vi "Scripting_UpdateGoop2Create.vi"(0 "ViRef":refnum<vi>, 1 "RemovePreloadDynamicMethods":bool, 5 "error in (no error)":errorcluster) -> (19 "error out":errorcluster)   [LabVIEW 2020]
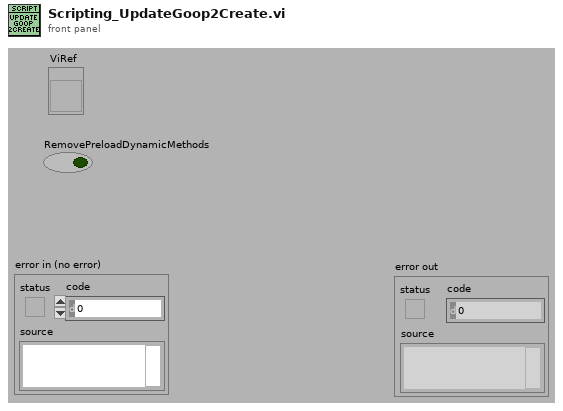
[diagram p1: front panel]
types:
  T1 = cluster{"OORefControls":refnum<vi>[], "ClassOORefs":path[], "ParentClassCreateVI":path}
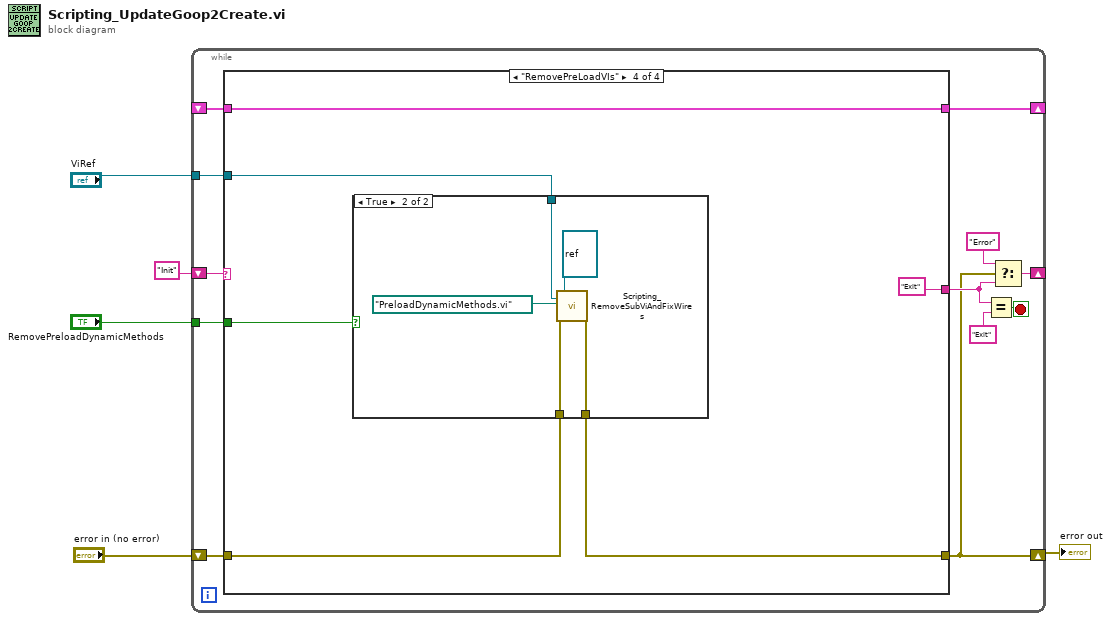
[diagram p0: block diagram]
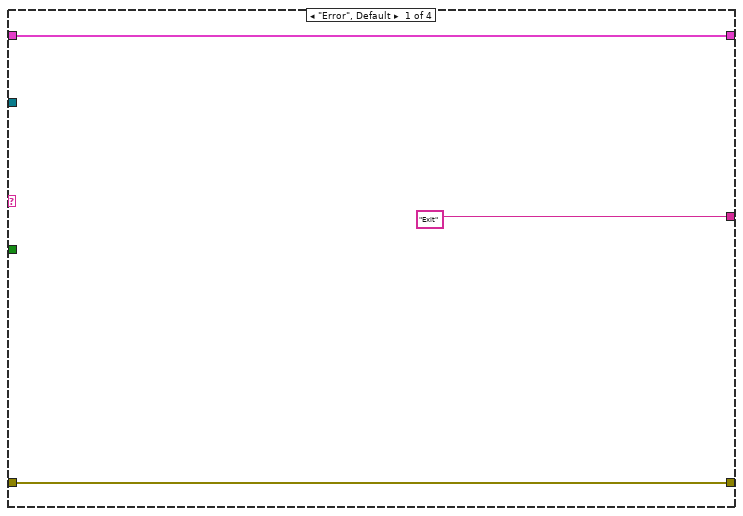
[diagram p2: hidden frame]
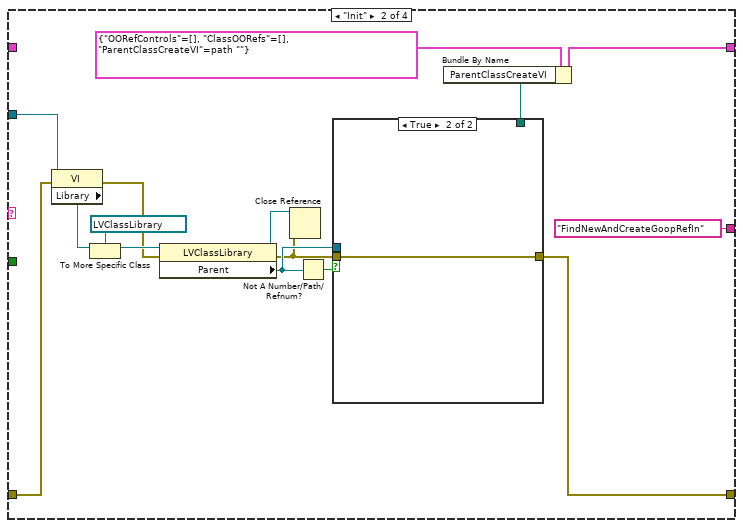
[diagram p3: hidden frame]
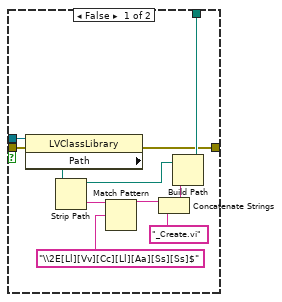
[diagram p4: hidden frame]
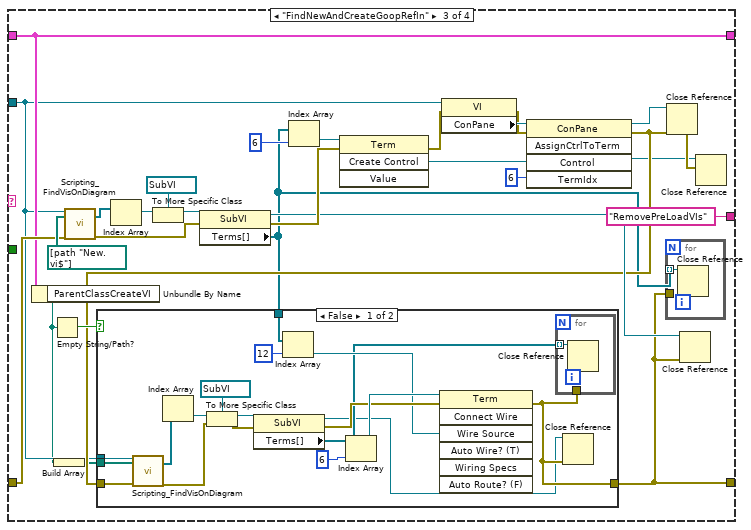
[diagram p5: hidden frame]
diagram:
  n1 = while {
    shift-right: [w10] -> w3
    shift-left: "error in (no error)" -> [w17]
    shift-right: [w15] -> _
    shift-left: "Init" -> [w16]
    shift-right: [w9] -> _
    shift-left: _ -> [w8]
    tunnel: "ViRef" -> [w7]
    tunnel: "RemovePreloadDynamicMethods" -> [w6]
    stop <- w14 stop-if-true
    n2 = case shown="\"RemovePreLoadVIs\"" w16 {
      tunnel: w17 -> [w20 w32 w59 w101]
      tunnel: [w20 w21 w55 w99] -> w10
      tunnel: ["Exit" "FindNewAndCreateGoopRefIn" "RemovePreLoadVIs" "Exit"] -> w11
      tunnel: [w18 w26 w58 w98] -> w9
      tunnel: w8 -> [w18 _ w58 w98]
      tunnel: w7 -> [_ w34 w53 w100]
      tunnel: w6 -> [_ _ _ w96]
      frame "Error", Default {
      }
      frame "Init" {
        n3 = property class="VI"(reference=w34, error in=w32) -> (error out=w28:errorcluster, "Library"=w31:refnum<vi>)  [unwired: 1 out]
        n4 = To More Specific Class(target class=refnum<vi> refnum ("LVClassLibrary Refnum"), reference=w31) -> (specific class reference=w29:refnum<vi>)  [unwired: 1 in, 1 out]
        n5 = property class="LVClassLibrary"(reference=w29, error in=w28) -> (reference out=w23:refnum<vi>, error out=w24:errorcluster, "Parent"=w25:refnum<vi>)
        n6 = Close Reference(reference=w23, error in (no error)=w24) -> ()  [unwired: 1 out]
        n7 = Not A Number/Path/Refnum?(number/path/refnum=w25) -> (NaN/Path/Refnum?=w33:bool)
        n8 = case shown="True" w33 {
          tunnel: w24 -> [w46 w47]
          tunnel: w25 -> [w45 _]
          tunnel: [w37 _] -> w22
          tunnel: [w36 w47] -> w21
          frame False {
            n9 = property class="LVClassLibrary"(reference=w45, error in=w46) -> (error out=w36:errorcluster, "Path"=w44:path)  [unwired: 1 out]
            n10 = Strip Path(path=w44) -> (stripped path=w38:path, name=w42:string)
            n11 = Match Pattern(string=w42, regular expression="\\2E[Ll][Vv][Cc][Ll][Aa][Ss][Ss]$") -> (before substring=w41:string)  [unwired: 1 in, 3 out]
            n12 = Concatenate Strings(w41, "_Create.vi" ("string")) -> (w39:string)
            n13 = Build Path(base path=w38, name or relative path=w39) -> (appended path=w37:path)
          }
          frame True {
          }
        }
        n14 = Bundle By Name(cluster=T1 {"OORefControls"=[], "ClassOORefs"=[], "ParentClassCreateVI"=path ""}, "ParentClassCreateVI"=w22) -> (w26:T1)
      }
      frame "FindNewAndCreateGoopRefIn" {
        n15 = Unbundle By Name(w58) -> ("ParentClassCreateVI"=w52:path)
        n16 = Empty String/Path?(string/path=w52) -> (empty?=w57:bool)
        n17 = Build Array(w52) -> (w51:path[])
        n18 = call "Scripting_FindVisOnDiagram.vi"("ViRef"=w53, "VIsToSerachFor/ViName"=path[] [path "New.vi$"] ("VIsToSerachFor"), "error in (no error)"=w59) -> ("VisFound"=w73:refnum<vi>[], "error out"=w69:errorcluster)  [unwired: 15 in]
        n19 = Index Array(array=w73) -> (element=w72:refnum<vi>)  [unwired: 1 in]
        n20 = To More Specific Class(target class=refnum<vi> refnum ("WhileLoop"), reference=w72) -> (specific class reference=w70:refnum<vi>)  [unwired: 1 in, 1 out]
        n21 = property class="SubVI"(reference=w70, error in=w69) -> (reference out=w60:refnum<vi>, error out=w66:errorcluster, "Terms[]"=w54:refnum<vi>[])
        n22 = Index Array(array=w54, index=6) -> (element=w67:refnum<vi>)
        n23 = invoke class="Term" method="Create Control"(reference=w67, error in=w66) -> (error out=w65:errorcluster, "Create Control"=w48:refnum<vi>)  [unwired: 2 in, 2 out]
        n24 = property class="VI"(reference=w53, error in=w65) -> (error out=w62:errorcluster, "ConPane"=w64:refnum<vi>)  [unwired: 1 out]
        n25 = invoke class="ConPane" method="AssignCtrlToTerm"(reference=w64, error in=w62, "Control"=w48, "TermIdx"=6 ("index")) -> (reference out=w61:refnum<vi>, error out=w56:errorcluster)  [unwired: 1 in, 3 out]
        n26 = case shown="False" w57 {
          tunnel: w56 -> [w92 w94]
          tunnel: [w76 w94] -> w55
          tunnel: w54 -> [w91 _]
          tunnel: w53 -> [w89 _]
          tunnel: w51 -> [w88 _]
          frame False {
            n27 = call "Scripting_FindVisOnDiagram.vi"("ViRef"=w89, "VIsToSerachFor/ViName"=w88, "error in (no error)"=w92) -> ("VisFound"=w87:refnum<vi>[], "error out"=w83:errorcluster)  [unwired: 15 in]
            n28 = Index Array(array=w87) -> (element=w84:refnum<vi>)  [unwired: 1 in]
            n29 = To More Specific Class(target class=refnum<vi> refnum ("WhileLoop"), reference=w84, error in=w83) -> (specific class reference=w86:refnum<vi>, error out=w79:errorcluster)
            n30 = property class="SubVI"(reference=w86, error in=w79) -> (reference out=w75:refnum<vi>, error out=w80:errorcluster, "Terms[]"=w77:refnum<vi>[])
            n31 = Index Array(array=w91, index=12) -> (element=w78:refnum<vi>)
            n32 = Index Array(array=w77, index=6) -> (element=w81:refnum<vi>)
            n33 = invoke class="Term" method="Connect Wire"(reference=w81, error in=w80, "Wire Source"=w78) -> (error out=w76:errorcluster)  [unwired: 4 in, 6 out]
            n34 = for {
              tunnel: w77 -> [w93] mode=indexing
              tunnel: w76 -> [_]
              n35 = Close Reference(reference=w93) -> ()  [unwired: 1 in, 1 out]
            }
            n36 = Close Reference(reference=w75, error in (no error)=w76) -> ()  [unwired: 1 out]
          }
          frame True {
          }
        }
        n37 = for {
          tunnel: w55 -> [_]
          tunnel: w54 -> [w95] mode=indexing
          n38 = Close Reference(reference=w95) -> ()  [unwired: 1 in, 1 out]
        }
        n39 = Close Reference(reference=w61, error in (no error)=w56) -> (error out=w49:errorcluster)
        n40 = Close Reference(reference=w60, error in (no error)=w55) -> ()  [unwired: 1 out]
        n41 = Close Reference(reference=w48, error in (no error)=w49) -> ()  [unwired: 1 out]
      }
      frame "RemovePreLoadVIs" {
        n42 = case shown="True" w96 {
          tunnel: w101 -> [w102 w106]
          tunnel: w100 -> [_ w105]
          tunnel: [w102 w104] -> w99
          frame False {
          }
          frame True {
            n43 = call "Scripting_RemoveSubViAndFixWires.vi"("MainViPath/ViRef/BlockDiagramRef"=w105, "SubVIToRemove"=path "PreloadDynamicMethods.vi" ("Path"), "error in (no error)"=w106, "AppRef"=refnum<vi> refnum) -> ("error out"=w104:errorcluster)  [unwired: 15 in]
          }
        }
      }
    }
    n44 = Equal?(x=w11, y="Exit") -> (x = y?=w14:bool)
    n45 = Select(t="Error", s=w10, f=w11) -> (s? t:f=w15:string)
  }
  "error out" <- w3
